vi "Fetch Measurement.vi"(8 "error in (no error)":errorcluster, 11 "DMM in":refnum<class "NI DMM.lvclass">) -> (0 "error out":errorcluster, 2 "Data":variant, 3 "DMM out":refnum<class "NI DMM.lvclass">)   [LabVIEW 2020, in "NI DMM.lvlib" / "NI DMM.lvclass"]
uses:
  NI DMM.lvclass
  NI DMM.lvclass/NI DMM.ctl
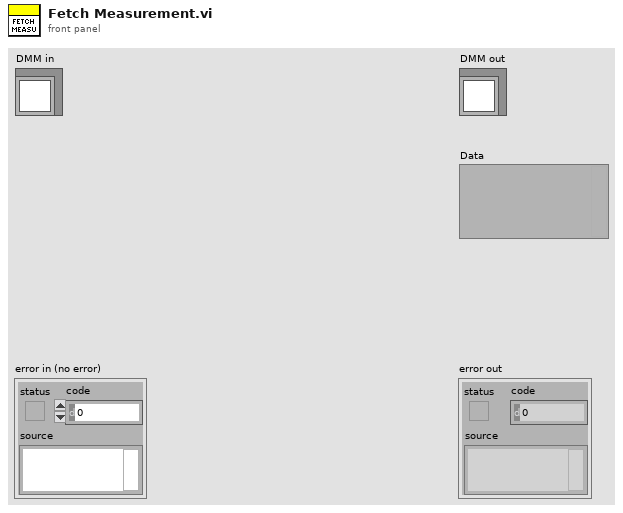
[diagram p1: front panel]
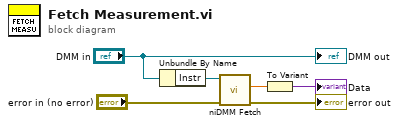
[diagram p0: block diagram]
diagram:
  n1 = Unbundle By Name("DMM in") -> ("Instr"=w5:refnum<k15>)
  n2 = call <instrlib>:"niDMM Fetch.vi"("error in (no error)"="error in (no error)", "instrument handle"=w5) -> ("error out"=→"error out":errorcluster, "Measurement"=w2:dbl)  [unwired: 7 in, 1 out]
  n3 = To Variant(anything=w2) -> (Variant=→"Data":variant)
  "DMM out" <- "DMM in"
